vi "Main_11b.vi"() -> ()   [LabVIEW 2021]
uses:
  4985a7b0-beb7-44e5-b21a-1b7cc2dea417.vi
  <vilib>/Comparison/Less/Less Functor/Less Functor.lvclass
panel:
  out "Post Round":T1(array[cluster])
  out "Answer":i32
  in  "Puzzle":string="Monkey 0:\n  Starting items: 72, 97\n  Operation: new = old * 13\n  Test: divisible by 19\n    If true: throw to monkey 5\n    If false: throw to monkey 6\n\nMonkey 1:\n  Starting items: 55, 70, 90, 74, 95\n  Operation: new = old * old\n  Test: divisible by 7\n    If true: throw to monkey 5\n    If false: throw to monkey 0\n\nMonkey 2:\n  Starting items: 74, 97, 66, 57\n  Operation: new = old + 6\n  Test: divisible by 17\n    If true: throw to monkey 1\n    If false: throw to monkey 0\n\nMonkey 3:\n  Starting items: 86, 54, 53\n  Operation: new = old + 2\n  Test: divisible by 13\n    If true: throw to monkey 1\n    If false: throw to monkey 2\n\nMonkey 4:\n  Starting items: 50, 65, 78, 50, 62, 99\n  Operation: new = old + 3\n  Test: divisible by 11\n    If true: throw to monkey 3\n    If false: throw to monkey 7\n\nMonkey 5:\n  Starting items: 90\n  Operation: new = old + 4\n  Test: divisible by 2\n    If true: throw to monkey 4\n    If false: throw to monkey 6\n\nMonkey 6:\n  Starting items: 88, 92, 63, 94, 96, 82, 53, 53\n  Operation: new = old + 8\n  Test: divisible by 5\n    If true: throw to monkey 4\n    If false: throw to monkey 7\n\nMonkey 7:\n  Starting items: 70, 60, 71, 69, 77, 70, 98\n  Operation: new = old * 7\n  Test: divisible by 3\n    If true: throw to monkey 2\n    If false: throw to monkey 3"
  in  "Example":string="Monkey 0:\n  Starting items: 79, 98\n  Operation: new = old * 19\n  Test: divisible by 23\n    If true: throw to monkey 2\n    If false: throw to monkey 3\n\nMonkey 1:\n  Starting items: 54, 65, 75, 74\n  Operation: new = old + 6\n  Test: divisible by 19\n    If true: throw to monkey 2\n    If false: throw to monkey 0\n\nMonkey 2:\n  Starting items: 79, 60, 97\n  Operation: new = old * old\n  Test: divisible by 13\n    If true: throw to monkey 1\n    If false: throw to monkey 3\n\nMonkey 3:\n  Starting items: 74\n  Operation: new = old + 3\n  Test: divisible by 17\n    If true: throw to monkey 0\n    If false: throw to monkey 1"
  # "15048718170"
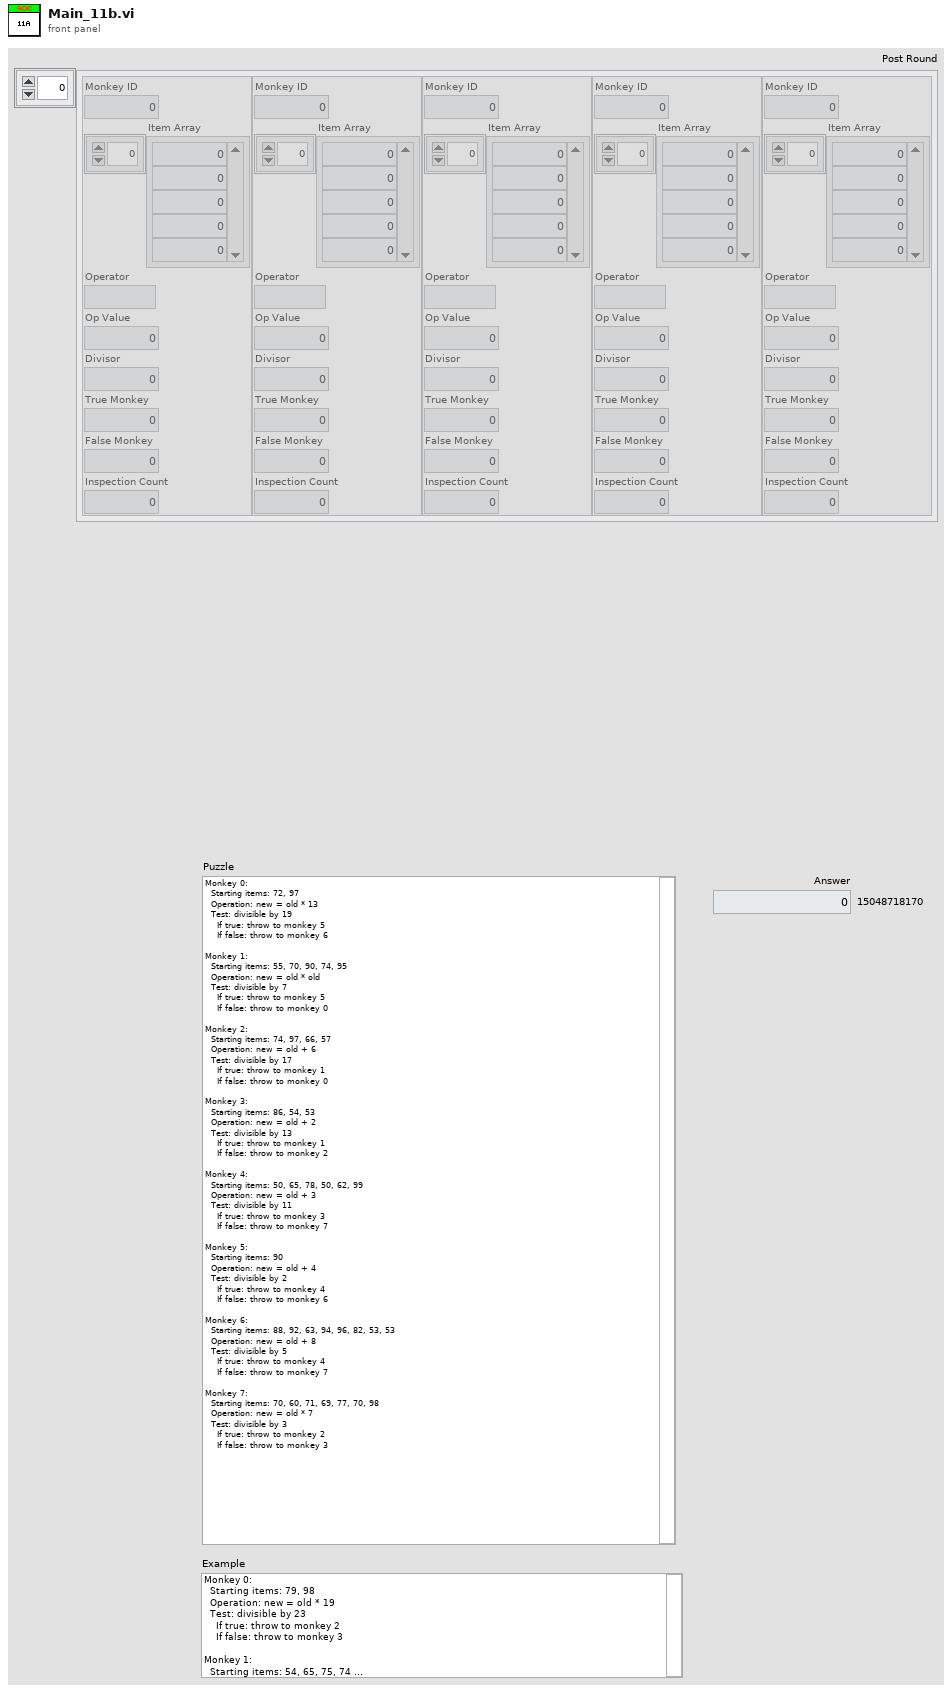
[diagram p1: front panel]
types:
  T1 = cluster{"Monkey ID":i32, "Item Array":i32[], "Operator":string, "Op Value":i32, "Divisor":i32, "True Monkey":i32, "False Monkey":i32, "Inspection Count":i32}[]
  T2 = cluster{"Monkey ID":i32, "Item Array":i32[], "Operator":string, "Op Value":i32, "Divisor":i32, "True Monkey":i32, "False Monkey":i32, "Inspection Count":i32}
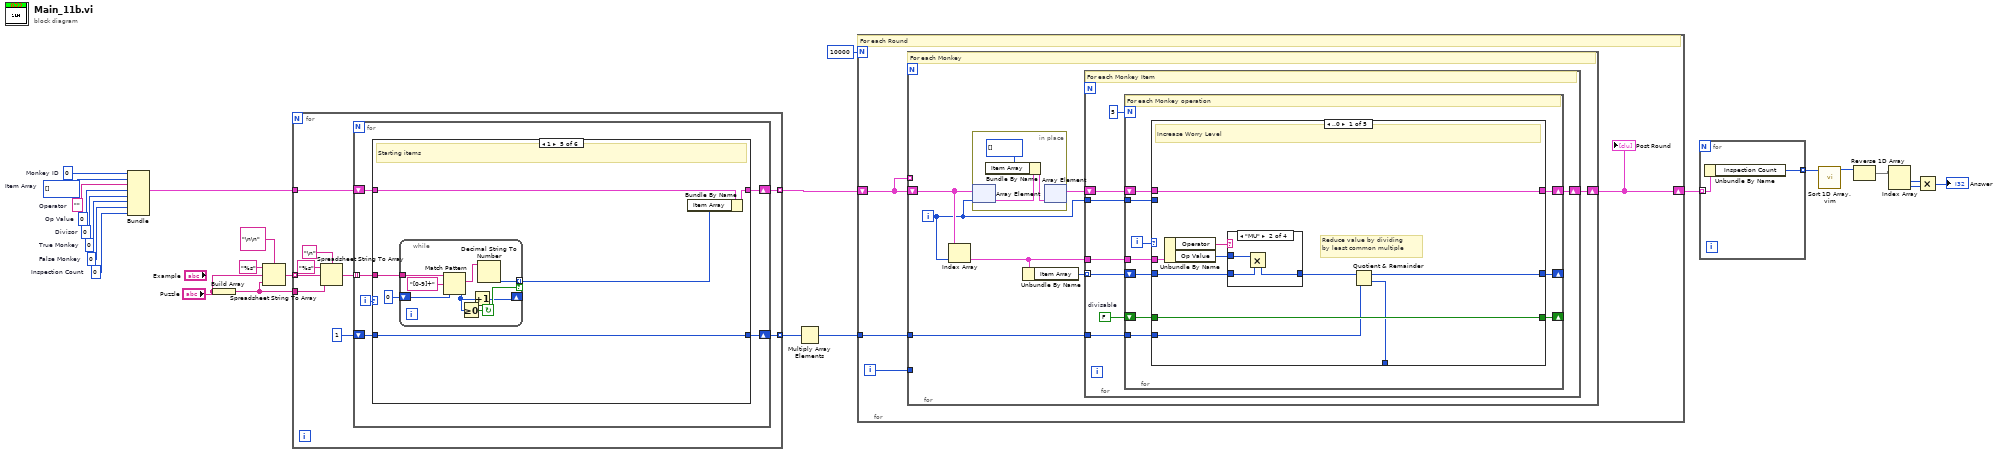
[diagram p0: block diagram]
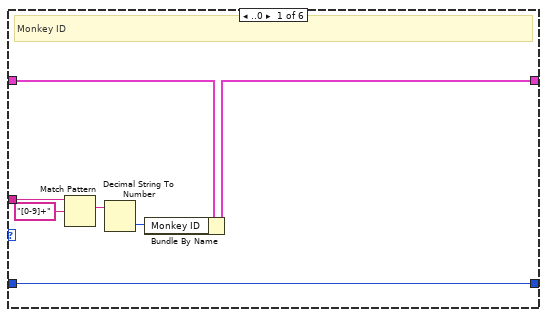
[diagram p2: hidden frame]
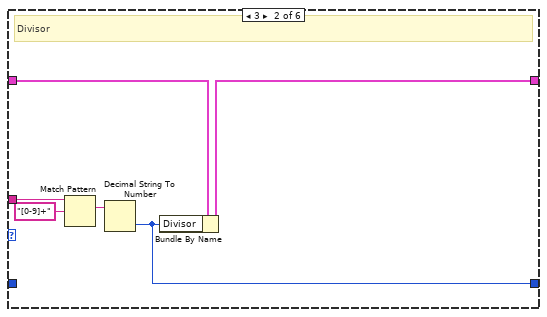
[diagram p3: hidden frame]
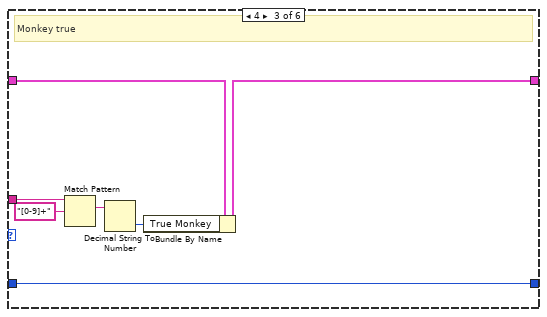
[diagram p4: hidden frame]
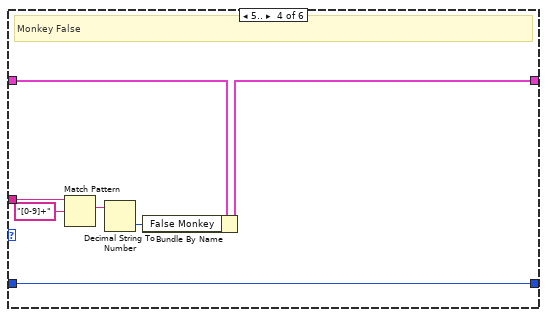
[diagram p5: hidden frame]
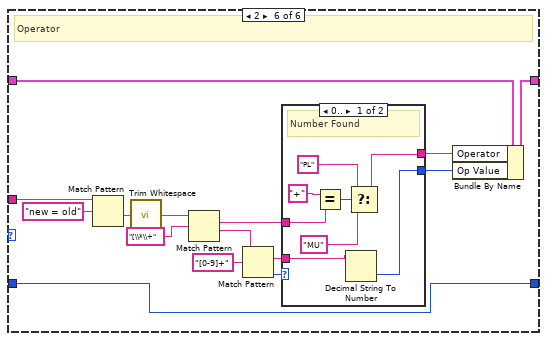
[diagram p6: hidden frame]
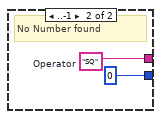
[diagram p7: hidden frame]
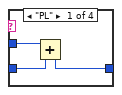
[diagram p8: hidden frame]
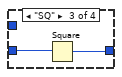
[diagram p9: hidden frame]
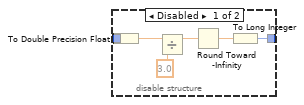
[diagram p12: hidden frame]
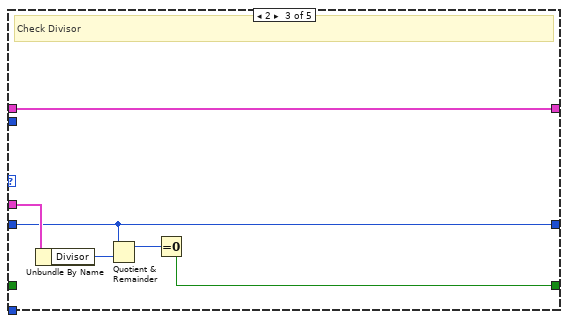
[diagram p13: hidden frame]
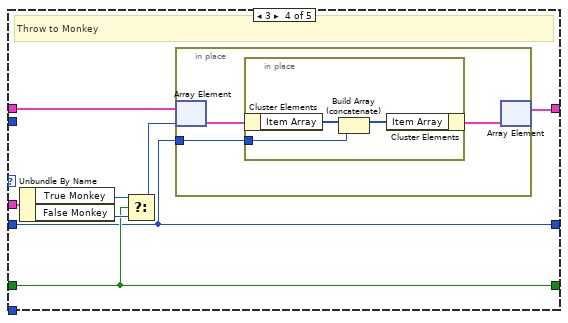
[diagram p14: hidden frame]
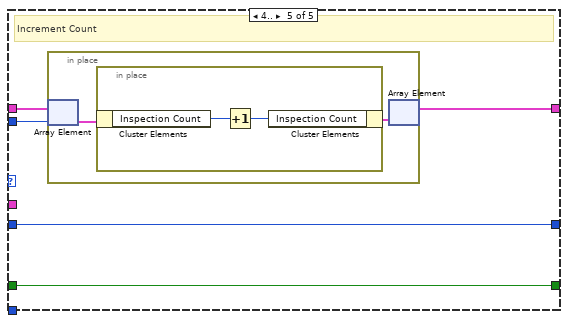
[diagram p15: hidden frame]
diagram:
  w11 = 0  # Inspection Count
  w14 = 0  # False Monkey
  w15 = 0  # True Monkey
  w16 = 0  # Divisor
  w17 = 0  # Op Value
  w18 = ""  # Operator
  w19 = i32[] []  # Item Array
  w20 = 0  # Monkey ID
  n1 = Bundle("Monkey ID"=w20, "Item Array"=w19, "Operator"=w18, "Op Value"=w17, "Divisor"=w16, "True Monkey"=w15, "False Monkey"=w14, "Inspection Count"=w11) -> (w13:T2)  [unwired: 1 in]
  n2 = Build Array("Puzzle") -> (w21:string[])
  n3 = Spreadsheet String To Array(delimiter (Tab)="\n\n", format string="%s", spreadsheet string="Puzzle", array type (2D Dbl)=w21) -> (array=w22:string[])
  n4 = for {
    tunnel: w22 -> [w34] mode=indexing
    tunnel: w21 -> [w31]
    tunnel: w13 -> [w29]
    tunnel: [w28] -> w12 mode=indexing
    tunnel: [w26] -> w2 mode=indexing
    n5 = Spreadsheet String To Array(delimiter (Tab)="\n", format string="%s", spreadsheet string=w34, array type (2D Dbl)=w31) -> (array=w30:string[])
    n6 = for {
      tunnel: w30 -> [w37] mode=indexing
      shift-right: [w38] -> w28
      shift-left: w29 -> [w39]
      shift-right: [w36] -> w26
      shift-left: 1 -> [w35]
      i -> [w40]
      n7 = case shown="1" w40 {
        tunnel: w39 -> [w47 w53 w60 w67 w73 w96]
        tunnel: [w46 w52 w59 w66 w72 w95] -> w38
        tunnel: w37 -> [w45 w51 w58 w65 w71 w94]
        tunnel: [w41 w48 w54 w61 w68 w82] -> w36
        tunnel: w35 -> [w41 _ w54 w61 w68 w82]
        frame ..0 {
          # "Monkey ID"
          n8 = Match Pattern(string=w45, regular expression="[0-9]+") -> (match substring=w43:string)  [unwired: 1 in, 3 out]
          n9 = Decimal String To Number(string=w43) -> (number=w42:i32)  [unwired: 2 in, 1 out]
          n10 = Bundle By Name(cluster=w47, "Monkey ID"=w42) -> (w46:T2)
        }
        frame 3 {
          # "Divisor"
          n11 = Match Pattern(string=w51, regular expression="[0-9]+") -> (match substring=w49:string)  [unwired: 1 in, 3 out]
          n12 = Decimal String To Number(string=w49) -> (number=w48:i32)  [unwired: 2 in, 1 out]
          n13 = Bundle By Name(cluster=w53, "Divisor"=w48) -> (w52:T2)
        }
        frame 4 {
          # "Monkey true"
          n14 = Match Pattern(string=w58, regular expression="[0-9]+") -> (match substring=w56:string)  [unwired: 1 in, 3 out]
          n15 = Decimal String To Number(string=w56) -> (number=w55:i32)  [unwired: 2 in, 1 out]
          n16 = Bundle By Name(cluster=w60, "True Monkey"=w55) -> (w59:T2)
        }
        frame 5.. {
          # "Monkey False"
          n17 = Match Pattern(string=w65, regular expression="[0-9]+") -> (match substring=w63:string)  [unwired: 1 in, 3 out]
          n18 = Decimal String To Number(string=w63) -> (number=w62:i32)  [unwired: 2 in, 1 out]
          n19 = Bundle By Name(cluster=w67, "False Monkey"=w62) -> (w66:T2)
        }
        frame 1 {
          # "Starting items"
          n20 = while {
            tunnel: w71 -> [w81]
            tunnel: [w77] -> w70 mode=indexing if=w79
            shift-right: [w75] -> _
            shift-left: 0 -> [w74]
            stop <- w79 continue-if-true
            n21 = Match Pattern(string=w81, regular expression="[0-9]+", offset (0)=w74) -> (match substring=w78:string, offset past match=w76:i32)  [unwired: 2 out]
            n22 = Greater Or Equal To 0?(x=w76) -> (x >= 0?=w79:bool)
            n23 = Increment(x=w76) -> (x+1=w75:i32)
            n24 = Decimal String To Number(string=w78) -> (number=w77:i32)  [unwired: 2 in, 1 out]
          }
          n25 = Bundle By Name(cluster=w73, "Item Array"=w70) -> (w72:T2)
        }
        frame 2 {
          # "Operator"
          n26 = Match Pattern(string=w94, regular expression="new = old") -> (after substring=w92:string)  [unwired: 1 in, 3 out]
          n27 = call <vilib>:"Trim Whitespace.vi"("string"=w92) -> ("trimmed string"=w90:string)  [unwired: 1 in]
          n28 = Match Pattern(string=w90, regular expression="[\\*\\+") -> (match substring=w84:string, after substring=w89:string)  [unwired: 1 in, 2 out]
          n29 = Match Pattern(string=w89, regular expression="[0-9]+") -> (match substring=w83:string, offset past match=w87:i32)  [unwired: 1 in, 2 out]
          n30 = case shown="0.." w87 {
            tunnel: [w99 w106] -> w86
            tunnel: [w97 0] -> w85
            tunnel: w84 -> [w103 _]
            tunnel: w83 -> [w98 _]
            frame 0.. {
              # "Number Found"
              n31 = Equal?(x="+", y=w103) -> (x = y?=w102:bool)
              n32 = Decimal String To Number(string=w98) -> (number=w97:i32)  [unwired: 2 in, 1 out]
              n33 = Select(t="PL", s=w102, f="MU") -> (s? t:f=w99:string)
            }
            frame ..-1 {
              w106 = "SQ"  # Operator
              # "No Number found"
            }
          }
          n34 = Bundle By Name(cluster=w96, "Operator"=w86, "Op Value"=w85) -> (w95:T2)
        }
      }
    }
  }
  n35 = Multiply Array Elements(1:w2) -> (0:w1:i32)
  n36 = for {
    N: 10000 -> [_]
    shift-right: [w109] -> w10
    shift-left: w12 -> [w110]
    tunnel: w1 -> [w108]
    i -> [w107]
    # "For each Round"
    n37 = for {
      shift-right: [w117] -> w109
      shift-left: w110 -> [w114]
      tunnel: w110 -> [_] mode=indexing
      tunnel: w108 -> [w111]
      tunnel: w107 -> [_]
      i -> [w113]
      # "For each Monkey"
      n38 = Index Array(array=w114, index=w113) -> (element=w112:T2)
      n39 = in-place {
        n40 = in-place-array #1(w114, w113) -> (w120:T2)
        n41 = Bundle By Name(cluster=w120, "Item Array"=i32[] []) -> (w119:T2)
        n42 = in-place-array #1(w119) -> (w115:T1)  [unwired: 1 out]
      }
      n43 = Unbundle By Name(w112) -> ("Item Array"=w116:i32[])
      n44 = for {
        tunnel: w112 -> [w126]
        tunnel: w116 -> [w127] mode=indexing
        shift-right: [w122] -> w117
        shift-left: w115 -> [w125]
        tunnel: w113 -> [w123]
        tunnel: w111 -> [w121]
        w124 = FALSE  # divisable
        # "For each Monkey Item"
        n45 = for {
          N: 5 -> [_]
          shift-right: [w134] -> _
          shift-left: w127 -> [w137]
          tunnel: w126 -> [w136]
          shift-right: [w133] -> w122
          shift-left: w125 -> [w135]
          shift-right: [w131] -> _
          shift-left: w124 -> [w132]
          tunnel: w123 -> [w130]
          tunnel: w121 -> [w129]
          i -> [w138]
          # "For each Monkey operation"
          n46 = case shown="..0" w138 {
            tunnel: w137 -> [w145 w161 w169 w175 w189]
            tunnel: w136 -> [w148 _ w173 w182 _]
            tunnel: w135 -> [w143 w159 w174 w178 w192]
            tunnel: [w141 w160 w169 w175 w189] -> w134
            tunnel: [w143 w159 w174 w177 w191] -> w133
            tunnel: w132 -> [w142 w158 _ w179 w193]
            tunnel: [w142 w158 w170 w179 w193] -> w131
            tunnel: w130 -> [_ _ _ _ w190]
            tunnel: w129 -> [w140 _ _ _ _]
            tunnel: [w139 _ _ _ _] -> _
            frame ..0 {
              # "Reduce value by dividing\nby least common multiple"
              # "Increase Worry Level"
              n47 = Unbundle By Name(w148) -> ("Operator"=w147:string, "Op Value"=w146:i32)
              n48 = case shown="\"MU\"" w147 {
                tunnel: w146 -> [w151 w154 _ _]
                tunnel: w145 -> [w150 w153 w156 w157]
                tunnel: [w149 w152 w155 w157] -> w144
                frame "PL" {
                  n49 = Add(x=w151, y=w150) -> (x+y=w149:i32)
                }
                frame "MU" {
                  n50 = Multiply(x=w154, y=w153) -> (x*y=w152:i32)
                }
                frame "SQ" {
                  n51 = Square(x=w156) -> (x^2=w155:i32)
                }
                frame Default {
                }
              }
              n52 = Quotient & Remainder(x=w144, y=w140) -> (x-y*floor(x/y)=w141:i32, floor(x/y)=w139:i32)
            }
            frame 1 {
              # "Divide worry by 3"
              n53 = disable-structure shown="Enabled" {
                disable-tunnel: w161 -> [w167 w168]
                disable-tunnel: [w162 w168] -> w160
                frame Disabled {
                  n54 = To Double Precision Float(number=w167) -> (double precision float=w166:dbl)
                  n55 = Divide(x=w166, y=3.0) -> (x/y=w164:dbl)
                  n56 = Round Toward -Infinity(1:w164) -> (0:w163:dbl)
                  n57 = To Long Integer(number=w163) -> (32bit integer=w162:i32)
                }
                frame Enabled {
                  # "Do not reduce worry"
                }
              }
            }
            frame 2 {
              # "Check Divisor"
              n58 = Unbundle By Name(w173) -> ("Divisor"=w172:i32)
              n59 = Quotient & Remainder(x=w169, y=w172) -> (x-y*floor(x/y)=w171:i32)  [unwired: 1 out]
              n60 = Equal To 0?(x=w171) -> (x = 0?=w170:bool)
            }
            frame 3 {
              # "Throw to Monkey"
              n61 = Unbundle By Name(w182) -> ("True Monkey"=w181:i32, "False Monkey"=w180:i32)
              n62 = Select(t=w181, s=w179, f=w180) -> (s? t:f=w176:i32)
              n63 = in-place {
                in-place-border: w175 -> [w183]
                n64 = in-place-array #2(w178, w176) -> (w185:T2)
                n65 = in-place {
                  in-place-border: w183 -> [w187]
                  n66 = in-place-cluster #3(w185) -> ("Item Array"=w188:i32[])
                  n67 = Build Array (concatenate)(w188, w187) -> (w186:i32[])
                  n68 = in-place-cluster #3("Item Array"=w186) -> (w184:T2)
                }
                n69 = in-place-array #2(w184) -> (w177:T1)  [unwired: 1 out]
              }
            }
            frame 4.. {
              # "Increment Count"
              n70 = in-place {
                n71 = in-place-array #4(w192, w190) -> (w195:T2)
                n72 = in-place {
                  n73 = in-place-cluster #5(w195) -> ("Inspection Count"=w197:i32)
                  n74 = Increment(x=w197) -> (x+1=w196:i32)
                  n75 = in-place-cluster #5("Inspection Count"=w196) -> (w194:T2)
                }
                n76 = in-place-array #4(w194) -> (w191:T1)  [unwired: 1 out]
              }
            }
          }
        }
      }
    }
    "Post Round" <- w109
  }
  n77 = for {
    tunnel: w10 -> [w199] mode=indexing
    tunnel: [w198] -> w9 mode=indexing
    n78 = Unbundle By Name(w199) -> ("Inspection Count"=w198:i32)
  }
  n79 = call "Sort 1D Array.vim"("unsorted array"=w9) -> ("sorted array"=w8:i32[])  [unwired: 10 in]
  n80 = Reverse 1D Array(array=w8) -> (reversed array=w7:i32[])
  n81 = Index Array(array=w7) -> (element #1=w5:i32, element #2=w6:i32)  [unwired: 2 in]
  n82 = Multiply(x=w5, y=w6) -> (x*y=→"Answer":i32)
